vi "Read Test.vi"(8 "error in (no error)":errorcluster, 11 "Bus in":refnum<class "Bus.lvclass">) -> (0 "error out":errorcluster, 2 "Test":refnum<class "Test.lvclass">[](array[class]), 3 "Bus out":refnum<class "Bus.lvclass">)   [LabVIEW 2014, in "Bus.lvclass"]
uses:
  Bus.lvclass
  TestClass/Test.lvclass
  Bus.lvclass/Bus.ctl
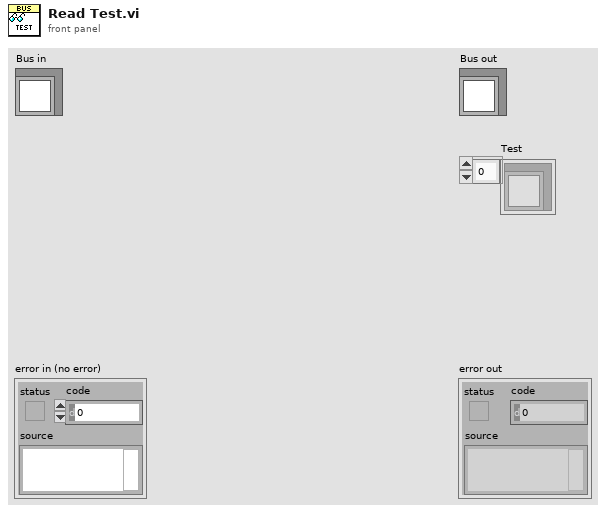
[diagram p1: front panel]
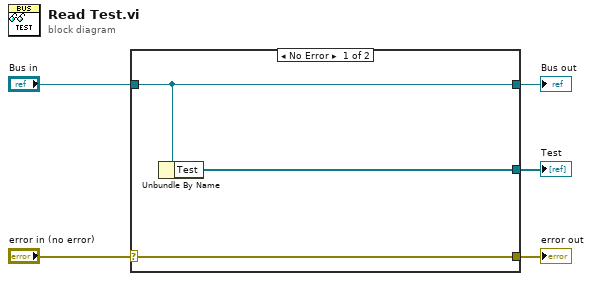
[diagram p0: block diagram]
diagram:
  n1 = case shown="No Error" "error in (no error)" {
    selector: "error in (no error)" -> [w8 w9]
    tunnel: [w8 w9] -> w4
    tunnel: [w7 w10] -> w2
    tunnel: "Bus in" -> [w7 w10]
    tunnel: [w6 _] -> w1
    frame No Error {
      n2 = Unbundle By Name(w7) -> ("Test"=w6:refnum<class "Test.lvclass">[])
    }
    frame Error {
    }
  }
  "error out" <- w4
  "Bus out" <- w2
  "Test" <- w1
